vi "_emi_S&E Q Generator.vi"(11 "error in (no error)":errorcluster) -> (8 "E&S Message Q":refnum<queue>, 15 "error out":errorcluster)   [LabVIEW 2011]
uses:
  _emi_ S&E Message.ctl
  _emi_ S&E Message type.ctl
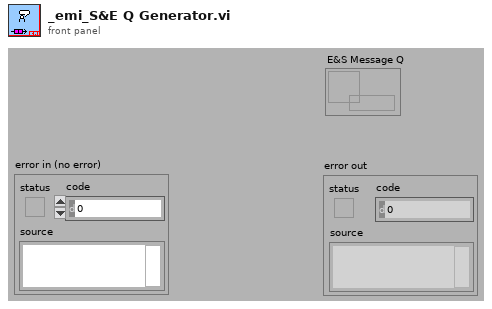
[diagram p1: front panel]
types:
  T1 = typedef "_emi_ S&E Message.ctl" = cluster{"Type":T2, "Originate time":dbl, "System":u8, "Loop":u16, "Sub ID":u16, "Elevated priority":bool, "E&S Message content":variant}
  T2 = typedef "_emi_ S&E Message type.ctl" = enum16{"Error/Warning", "Note", "Debug", "Event", "Alarm Analog", "Alarm Digital", "Annotation"}
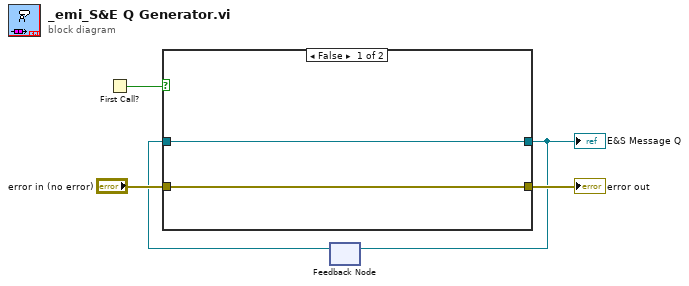
[diagram p0: block diagram]
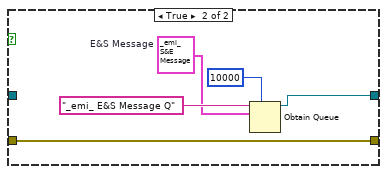
[diagram p2: hidden frame]
diagram:
  n1 = First Call?() -> (First Call?: T/F=w3:bool)
  n2 = feedback #1() -> (w1:refnum<queue>)  [unwired: 1 in]
  n3 = case shown="False" w3 {
    tunnel: [w7 w8] -> w5
    tunnel: "error in (no error)" -> [w7 w8]
    tunnel: [w6 w12] -> w2
    tunnel: w1 -> [w6 _]
    frame False {
    }
    frame True {
      w10 = T1 {"Type"=enum."Error/Warning", "Originate time"=0.0, "System"=0, "Loop"=0, "Sub ID"=0, "Elevated priority"=FALSE, "E&S Message content"=variant}  # E&S Message
      n4 = Obtain Queue(max queue size (-1, unlimited)=10000, name (unnamed)="_emi_ E&S Message Q", element data type=w10) -> (queue out=w12:refnum<queue>)  [unwired: 2 in, 2 out]
    }
  }
  "error out" <- w5
  "E&S Message Q" <- w2
  n5 = feedback-in #1(w2) -> ()
